vi "Practica_12_BInario a7 Segmentos.vi"() -> ()   [LabVIEW 2016]
panel:
  in  "Enum":T1(ring)
  out "Array":bool[](array[boolean])
  in  "Down Button":bool
  in  "Up Button":bool
  out "Segmento E":bool
  out "Segmento C":bool
  out "Segmento D":bool
  out "Segmendo G":bool
  out "Segmento B":bool
  out "Segmento F":bool
  out "Segmento A":bool
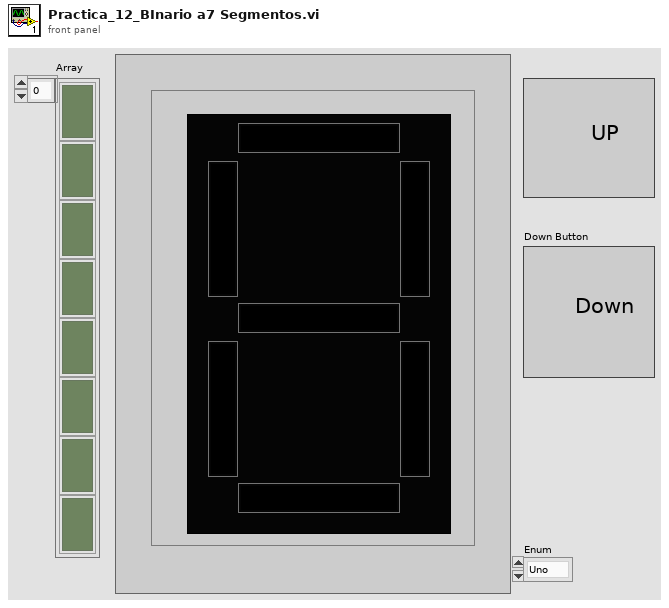
[diagram p1: front panel]
types:
  T1 = enum16{"Uno", "Dos", "Tres", "Cuatro", "Cinco", "Seis", "Siete", "Ocho", "Nueve", "Cero"}
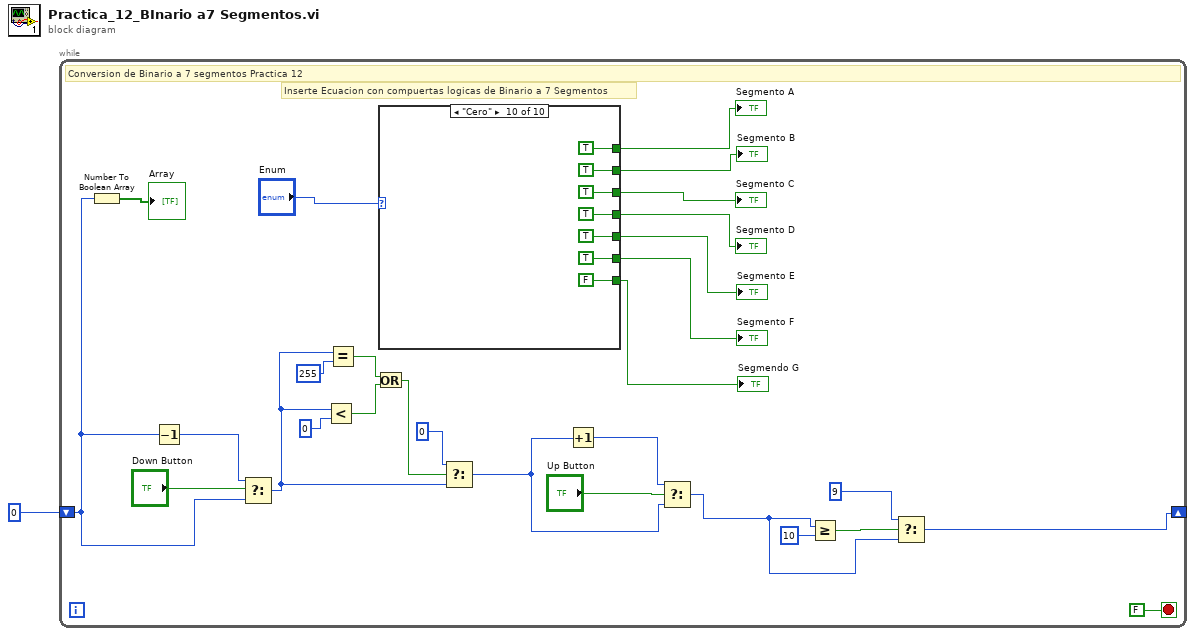
[diagram p0: block diagram]
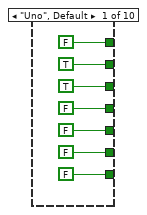
[diagram p2: hidden frame]
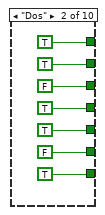
[diagram p3: hidden frame]
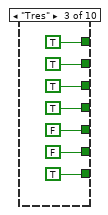
[diagram p4: hidden frame]
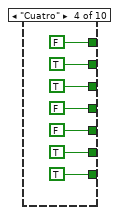
[diagram p5: hidden frame]
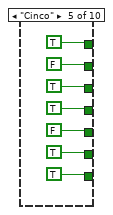
[diagram p6: hidden frame]
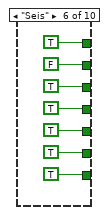
[diagram p7: hidden frame]
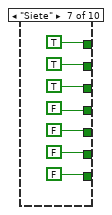
[diagram p8: hidden frame]
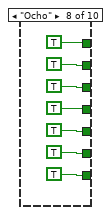
[diagram p9: hidden frame]
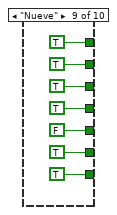
[diagram p10: hidden frame]
diagram:
  n1 = while {
    shift-right: [w21] -> _
    shift-left: u8 0 -> [w10]
    stop <- FALSE stop-if-true
    # "Inserte Ecuacion con compuertas logicas de Binario a 7 Segmentos"
    # "Conversion de Binario a 7 segmentos Practica 12"
    n2 = Number To Boolean Array(number=w10) -> (Boolean array=→"Array":bool[])
    n3 = Decrement(x=w10) -> (x-1=w26:u8)
    n4 = Select(t=w26, s="Down Button", f=w10) -> (s? t:f=w18:u8)
    n5 = Less?(x=w18, y=u8 0) -> (x < y?=w16:bool)
    n6 = Equal?(x=w18, y=u8 255) -> (x = y?=w15:bool)
    n7 = Or(x=w15, y=w16) -> (x .or. y?=w14:bool)
    n8 = case shown="\"Cero\"" "Enum" {
      tunnel: [FALSE TRUE TRUE FALSE TRUE TRUE TRUE TRUE TRUE TRUE] -> w8
      tunnel: [TRUE TRUE TRUE TRUE FALSE FALSE TRUE TRUE TRUE TRUE] -> w7
      tunnel: [TRUE FALSE TRUE TRUE TRUE TRUE TRUE TRUE TRUE TRUE] -> w6
      tunnel: [FALSE TRUE TRUE FALSE TRUE TRUE FALSE TRUE TRUE TRUE] -> w5
      tunnel: [FALSE TRUE FALSE FALSE FALSE TRUE FALSE TRUE FALSE TRUE] -> w4
      tunnel: [FALSE FALSE FALSE TRUE TRUE TRUE FALSE TRUE TRUE TRUE] -> w3
      tunnel: [FALSE TRUE TRUE TRUE TRUE TRUE FALSE TRUE TRUE FALSE] -> w2
      frame "Uno", Default {
      }
      frame "Dos" {
      }
      frame "Tres" {
      }
      frame "Cuatro" {
      }
      frame "Cinco" {
      }
      frame "Seis" {
      }
      frame "Siete" {
      }
      frame "Ocho" {
      }
      frame "Nueve" {
      }
      frame "Cero" {
      }
    }
    "Segmento A" <- w8
    "Segmento F" <- w3
    "Segmento B" <- w7
    "Segmendo G" <- w2
    "Segmento D" <- w5
    "Segmento C" <- w6
    "Segmento E" <- w4
    n9 = Select(t=u8 0, s=w14, f=w18) -> (s? t:f=w13:u8)
    n10 = Increment(x=w13) -> (x+1=w25:u8)
    n11 = Select(t=w25, s="Up Button", f=w13) -> (s? t:f=w12:u8)
    n12 = Greater Or Equal?(x=w12, y=u8 10) -> (x >= y?=w23:bool)
    n13 = Select(t=u8 9, s=w23, f=w12) -> (s? t:f=w21:u8)
  }
